vi "Set message.vi"(10 "WampMessage JSON":refnum<class "WampMessage JSON.lvclass">, 11 "IMsgPackMessageHandler in":refnum<class "ResultHandler JSON.lvclass">) -> (3 "IMsgPackMessageHandler out":refnum<class "ResultHandler JSON.lvclass">)   [LabVIEW 2020, in "wamplv.lvlib" / "ResultHandler JSON.lvclass"]
uses:
  ResultHandler JSON.lvclass
  ResultHandler JSON.lvclass/ResultHandler JSON.ctl
  SerialisedMessages/JSONMessage/WampMessage JSON.lvclass
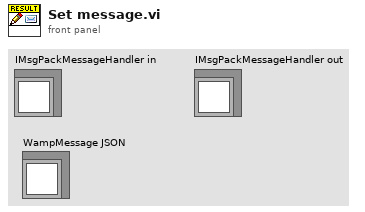
[diagram p1: front panel]
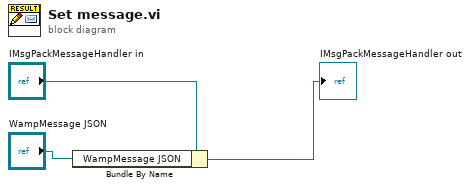
[diagram p0: block diagram]
diagram:
  n1 = Bundle By Name(cluster="IMsgPackMessageHandler in", "WampMessage JSON"="WampMessage JSON") -> (→"IMsgPackMessageHandler out":refnum<class "ResultHandler JSON.lvclass">)
